vi "SUB-BLE Rx data (Mon)-CDC IMU.vi"(8 "data in":u8[](array[numeric]) format="%2x") -> (0 "IMU data":T1 caption="IMU Monitoring data" {"Accelerometer Z" format="%#.9f"; "Accelerometer Y" format="%#.9f"; "Accelerometer X" format="%#.9f"; "Gyroscope Z" format="%#.9f"; "Gyroscope Y" format="%#.9f"; "Gyroscope X" format="%#.9f"}, 1 "CDC data":T2 caption="CDC Monitoring data" {"Right Wing-C, C6/C0" format="%#.9f"; "Right Wing-B, C5/C0" format="%#.9f"; "Right Wing-A, C4/C0" format="%#.9f"; "Left Wing-C, C3/C0" format="%#.9f"; "Left Wing-B, C2/C0" format="%#.9f"; "Left Wing-A, C1/C0" format="%#.9f"}, 2 "Bat":u16, 3 "*Board ID":string="None...." caption="S/N")   [LabVIEW 2015]
doc: "Use this template to create an application that executes repeatedly until you click the Stop button. This template polls the state of the Stop button and does not use events. Use the Top-Level Application template (not available in the Base package) to create a single-loop application with event handling."
uses:
  Control-CDC data.ctl
  Control-IMU data.ctl
panel:
  out "원소":u8
  out "BLE Packet (buf)":u8[](array[numeric])
  out "BLE Packet (data)":u8[](array[numeric])
  # "BLE 수신 데이터를 분류: Monitoring/Setting data"
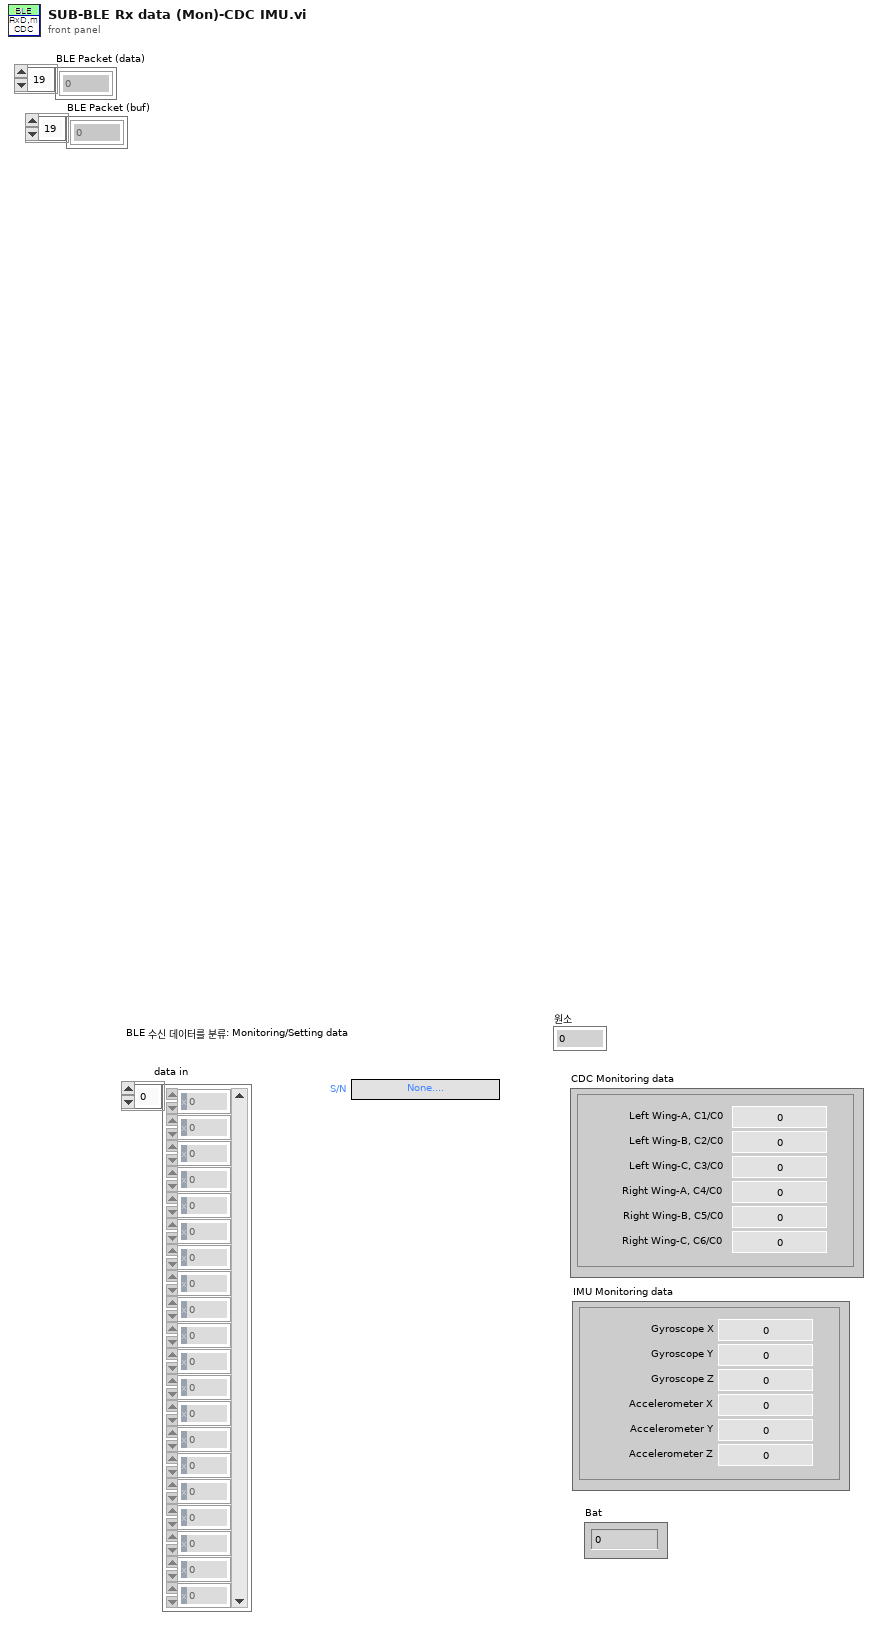
[diagram p1: front panel]
types:
  T1 = typedef "Control-IMU data.ctl" = cluster{"Gyroscope X":dbl, "Gyroscope Y":dbl, "Gyroscope Z":dbl, "Accelerometer X":dbl, "Accelerometer Y":dbl, "Accelerometer Z":dbl}
  T2 = typedef "Control-CDC data.ctl" = cluster{"Left Wing-A, C1/C0":dbl, "Left Wing-B, C2/C0":dbl, "Left Wing-C, C3/C0":dbl, "Right Wing-A, C4/C0":dbl, "Right Wing-B, C5/C0":dbl, "Right Wing-C, C6/C0":dbl}
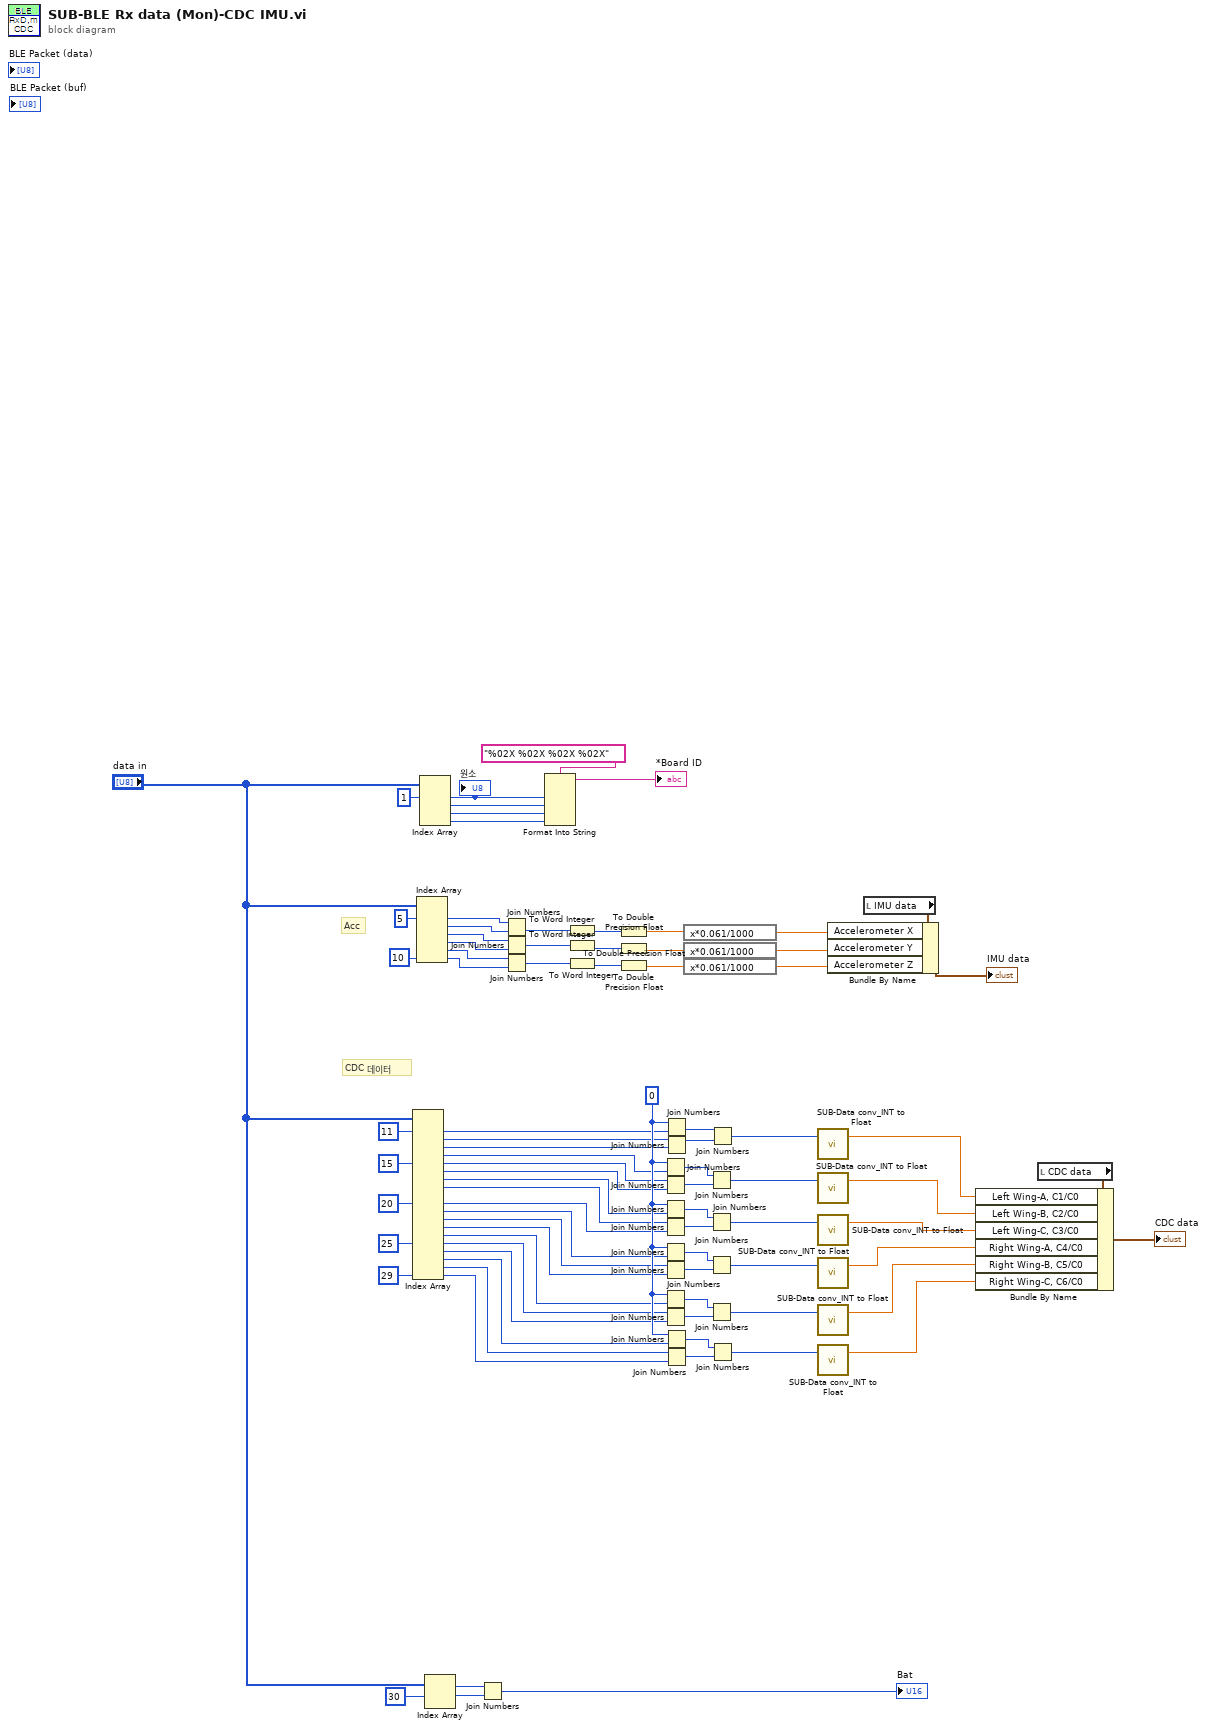
[diagram p0: block diagram]
diagram:
  w35 = u8 0 ("hi")
  # "Acc"
  # "CDC 데이터"
  n1 = Index Array(array="data in", index #1=11 ("인덱스"), index #5=15 ("인덱스"), index #10=20 ("인덱스"), index #15=25 ("인덱스"), index #19=29 ("인덱스")) -> (element #1=w34:u8, element #2=w33:u8, element #3=w32:u8, element #4=w31:u8, element #5=w30:u8, element #6=w29:u8, element #7=w28:u8, element #8=w27:u8, element #10=w22:u8, element #11=w21:u8, element #12=w20:u8, element #13=w19:u8, element #14=w18:u8, element #15=w17:u8, element #16=w16:u8, element #17=w15:u8, element #18=w14:u8, element #19=w13:u8)  [unwired: 14 in, 1 out]
  n2 = Index Array(array="data in", index #1=5 ("인덱스"), index #6=10 ("인덱스")) -> (element #1=w55:u8, element #2=w54:u8, element #3=w53:u8, element #4=w52:u8, element #5=w51:u8, element #6=w50:u8)  [unwired: 4 in]
  n3 = Index Array(array="data in", index #1=1 ("인덱스")) -> (element #1=w82:u8, element #2=w81:u8, element #3=w80:u8, element #4=w79:u8)  [unwired: 3 in]
  "원소" <- w82
  n4 = Index Array(array="data in", index #1=30 ("인덱스")) -> (element #1=w68:u8, element #2=w69:u8)  [unwired: 1 in]
  n5 = Join Numbers(hi=w68, lo=w69) -> ((hi.lo)=→"Bat":u16)
  n6 = Join Numbers(hi=w55, lo=w54) -> ((hi.lo)=w62:u16)
  n7 = Join Numbers(hi=w53, lo=w52) -> ((hi.lo)=w61:u16)
  n8 = Join Numbers(hi=w51, lo=w50) -> ((hi.lo)=w60:u16)
  n9 = Format Into String(format string="%02X %02X %02X %02X" ("구분 문자(탭)"), w82, w81, w80, w79) -> (resulting string=→"*Board ID":string)  [unwired: 2 in, 1 out]
  n10 = To Word Integer(number=w62) -> (16bit integer=w65:i16)
  n11 = To Word Integer(number=w61) -> (16bit integer=w64:i16)
  n12 = To Word Integer(number=w60) -> (16bit integer=w63:i16)
  n13 = To Double Precision Float(number=w65) -> (double precision float=w73:dbl)
  n14 = To Double Precision Float(number=w64) -> (double precision float=w72:dbl)
  n15 = To Double Precision Float(number=w63) -> (double precision float=w71:dbl)
  n16 = Join Numbers(hi=w35, lo=w31) -> ((hi.lo)=w45:u16)
  n17 = Join Numbers(hi=w30, lo=w29) -> ((hi.lo)=w44:u16)
  n18 = Join Numbers(hi=w35, lo=w28) -> ((hi.lo)=w42:u16)
  n19 = Join Numbers(hi=w27, lo=w22) -> ((hi.lo)=w43:u16)
  n20 = Join Numbers(hi=w35, lo=w21) -> ((hi.lo)=w41:u16)
  n21 = Join Numbers(hi=w20, lo=w19) -> ((hi.lo)=w40:u16)
  n22 = Join Numbers(hi=w35, lo=w18) -> ((hi.lo)=w38:u16)
  n23 = Join Numbers(hi=w17, lo=w16) -> ((hi.lo)=w39:u16)
  n24 = Join Numbers(hi=w35, lo=w34) -> ((hi.lo)=w46:u16)
  n25 = Join Numbers(hi=w33, lo=w32) -> ((hi.lo)=w47:u16)
  n26 = Join Numbers(hi=w35, lo=w15) -> ((hi.lo)=w37:u16)
  n27 = Join Numbers(hi=w14, lo=w13) -> ((hi.lo)=w36:u16)
  n28 = expression code="x*0.061/1000"(w73) -> (w58:dbl)
  n29 = expression code="x*0.061/1000"(w72) -> (w57:dbl)
  n30 = expression code="x*0.061/1000"(w71) -> (w56:dbl)
  n31 = Join Numbers(hi=w45, lo=w44) -> ((hi.lo)=w11:u32)
  n32 = Join Numbers(hi=w42, lo=w43) -> ((hi.lo)=w10:u32)
  n33 = Join Numbers(hi=w41, lo=w40) -> ((hi.lo)=w9:u32)
  n34 = Join Numbers(hi=w38, lo=w39) -> ((hi.lo)=w8:u32)
  n35 = Join Numbers(hi=w46, lo=w47) -> ((hi.lo)=w12:u32)
  n36 = Join Numbers(hi=w37, lo=w36) -> ((hi.lo)=w7:u32)
  n37 = call "SUB-Data conv_INT to Float.vi"("U32"=w12) -> ("FP32"=w6:sgl)  [unwired: 2 in]
  n38 = call "SUB-Data conv_INT to Float.vi"("U32"=w11) -> ("FP32"=w5:sgl)  [unwired: 2 in]
  n39 = call "SUB-Data conv_INT to Float.vi"("U32"=w10) -> ("FP32"=w4:sgl)  [unwired: 2 in]
  n40 = call "SUB-Data conv_INT to Float.vi"("U32"=w9) -> ("FP32"=w3:sgl)  [unwired: 2 in]
  n41 = call "SUB-Data conv_INT to Float.vi"("U32"=w8) -> ("FP32"=w2:sgl)  [unwired: 2 in]
  n42 = call "SUB-Data conv_INT to Float.vi"("U32"=w7) -> ("FP32"=w1:sgl)  [unwired: 2 in]
  n43 = local read "IMU data"() -> (w74:T1)
  n44 = Bundle By Name(cluster=w74, "Accelerometer X"=w58, "Accelerometer Y"=w57, "Accelerometer Z"=w56) -> (→"IMU data":T1)
  n45 = local read "CDC data"() -> (w77:T2)
  n46 = Bundle By Name(cluster=w77, "Left Wing-A, C1/C0"=w6, "Left Wing-B, C2/C0"=w5, "Left Wing-C, C3/C0"=w4, "Right Wing-A, C4/C0"=w3, "Right Wing-B, C5/C0"=w2, "Right Wing-C, C6/C0"=w1) -> (→"CDC data":T2)
